vi "确认表格插入位置.vi"(10 "Cpk计算数量":i32, 11 "MS Office parameters out":T1) -> (1 "position (Excel)":cluster{"row":i32, "column":i32}, 2 "簇":cluster{"row":i32, i32}, 3 "簇 2":cluster{"f":i32, i32}, 4 "起始":cluster{i32, i32}, 5 "结束行":cluster{"row":i32, "column":i32})   [LabVIEW 2014]
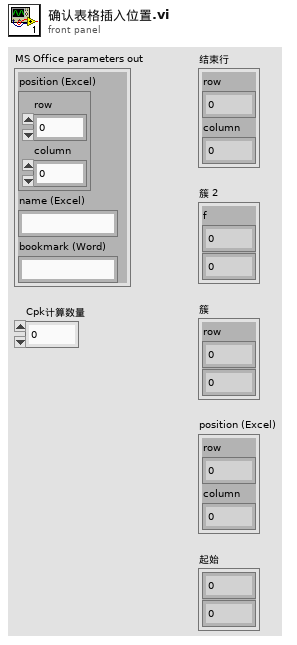
[diagram p1: front panel]
types:
  T1 = cluster{"position (Excel)":cluster{"row":i32, "column":i32}, "name (Excel)":string, "bookmark (Word)":string}
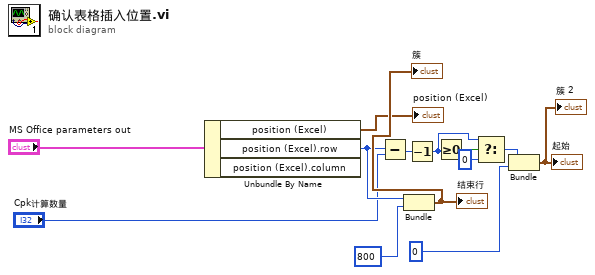
[diagram p0: block diagram]
diagram:
  n1 = Unbundle By Name("MS Office parameters out") -> ("position (Excel)"=→"position (Excel)":cluster{"row":i32, "column":i32}, "position (Excel).row"=w11:i32)  [unwired: 1 out]
  n2 = Subtract(x=w11, y="Cpk计算数量") -> (x-y=w2:i32)
  n3 = Bundle("row"=w11, 800) -> (→"结束行" →"簇":cluster{"row":i32, i32})  [unwired: 1 in]
  n4 = Decrement(x=w2) -> (x-1=w8:i32)
  n5 = Greater Or Equal To 0?(x=w8) -> (x >= 0?=w7:bool)
  n6 = Select(t=w8, s=w7, f=0) -> (s? t:f=w10:i32)
  n7 = Bundle("f"=w10, 0) -> (→"起始" →"簇 2":cluster{"f":i32, i32})  [unwired: 1 in]
